vi "tsapp_add_application.vi"(8 "error in (no error)":errorcluster caption="错误输入（无错误）", 10 "AAppName":string, 11 "路径输入":path) -> (0 "error out":errorcluster caption="错误输出", 2 "retuen":i32, 3 "路径输出":path)   [LabVIEW 2014]
doc: "Function Introduction ：\nAdd applications by name, after which you can add or edit channel mappings\nCall location ：\nBefore the start of the application lifecycle\ninput parameter ：\nAAppName: Program Name\nReturn value ：\n==0: Execution successful\nOther results: Query error code"
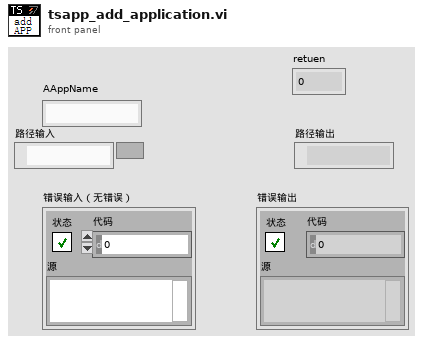
[diagram p1: front panel]
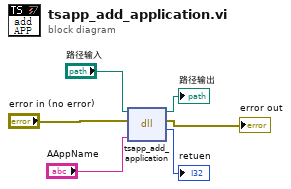
[diagram p0: block diagram]
diagram:
  n1 = dll-call lib="D:/Work/LabVIEW Code/TSMaster Labview SDK/LabVIEW/LabVIEW-TSMasterAPI_CLN/TSMasterAPI_LabVIEW-2024-08-02 09-14-06/Not_organized_vi/TSMaster.*" fn="tsapp_add_application"(path in="路径输入", error in="error in (no error)", "AAppName"="AAppName") -> (path out=→"路径输出":path, error out=→"error out":errorcluster, "返回类型"=→"retuen":i32)  [unwired: 2 in]
